vi "get_fifo.vi"(11 "FIFO":string) -> (1 "XY Graph":cluster{i32[], dbl[]}[](graph), 3 "Array":T2(array[cluster]))   [LabVIEW 2020]
panel:
  out "x/y":cdb[](array[numeric])
  out "Waveform Graph":i32[](graph)
  out "value":T1
  out "Cluster":T1
  out "rest of the binary string":string
  out "Numeric 2":u16
  in  "Numeric":u16 format="%x"
  out "Array 4":i32[](array[numeric])
  out "length 2":i32
  out "data string":string
  out "offset (0)":i32=31
  out "read buffer":string
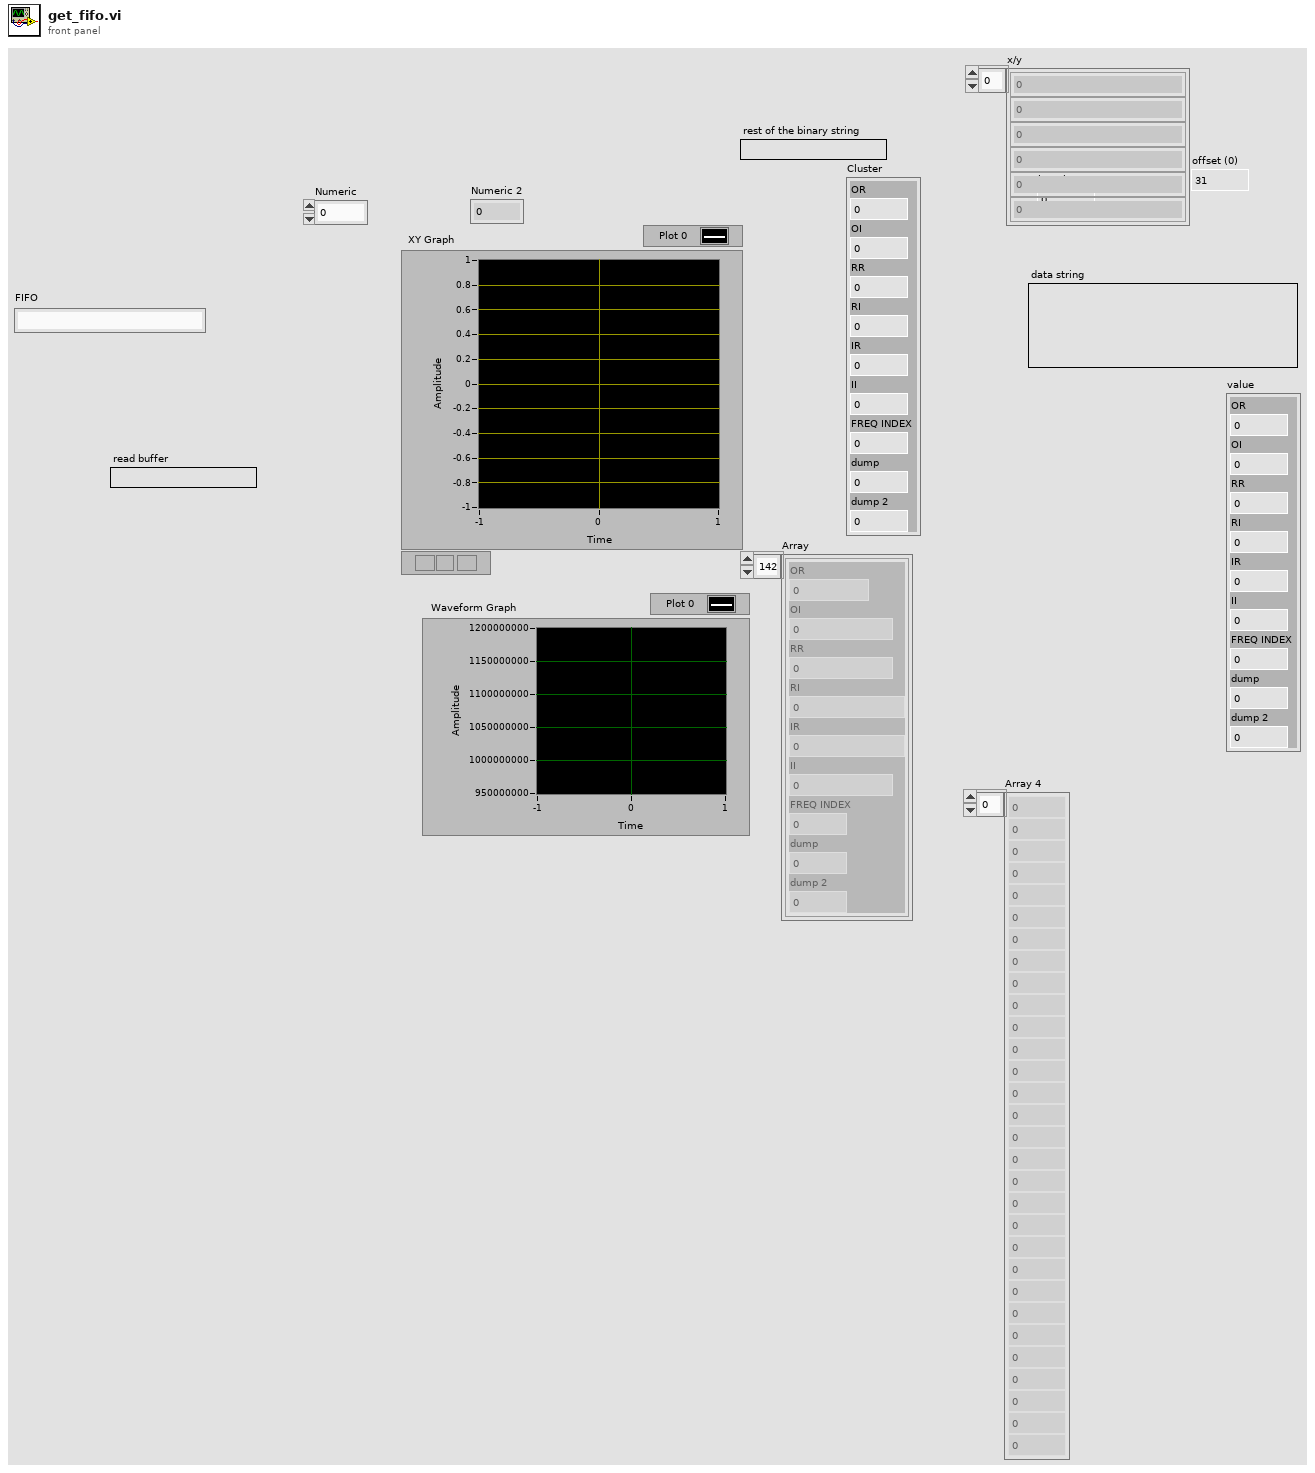
[diagram p1: front panel]
types:
  T1 = cluster{"OR":i32, "OI":i32, "RR":i32, "RI":i32, "IR":i32, "II":i32, "FREQ INDEX":u16, "dump":u16, "dump 2":u32}
  T2 = cluster{"OR":i32, "OI":i32, "RR":i32, "RI":i32, "IR":i32, "II":i32, "FREQ INDEX":u16, "dump":u16, "dump 2":u32}[]
  T3 = enum16{"big-endian, network order", "native, host order", "little-endian"}
diagram:
  w2 = 32 ("offset (0)")
  (unwired) "\u0000\u0000\u0000@\u0000\u0000\u0000\u0000l\u0002I\u0014Ü\b\u0000\u0000\u0000ÿÿÿ\u0001\u0000\u0000\u0000\u0000\u0000\u0000y\u0000\u0000\u0000@\u0000\u0000\u0000\u0000\u0006²ð/aFÿÿÿÿÿÿ\u0001\u0000\u0000\u0000\u0000\u0000\u0000Â\u0000\u0000\u0000@\u0000\u0000\u0000\u0000\u0000C!ÅP\u0000\u0000\u0000ÿÿÿ\u0001\u0000\u0000\u0000\u0000\u0000\u0000E\u0000\u0000\u0000@\u0000\u0000\u0000\u0000àb%\u001f¸£ùÿÿÿ\u0000\u0000\u0000\u0001\u0000\u0000\u0000\u0000\u0000\u0000\u0000\u0000\u0000@\u0000\u0000\u0000\u0000 y[ò@¹\u0007>\u0000\u0000\u0000\u0000\u0000\u0000\u0001\u0000\u0000\u0000\u0000\u0000\u0000p\u0000\u0000\u0000@\u0000\u0000\u0000\u0000\u0000 ÆD\u0000Üe\u0000\u0000\u0000\u0000\u0000\u0000\u0001\u0000\u0000\u0000\u0000\u0000\u0000k\u0000\u0000\u0000@\u0000\u0000\u0000\u0000 \\\u0010ðGÍ\u0001\u0000\u0000\u0000ÿÿÿ\u0001\u0000\u0000\u0000\u0000\u0000\u0000>\u0000\u0000\u0000@\u0000\u0000\u0000\u0000Ð\u0003¬\u0007ÿÿÿ\u0000\u0000\u0000\u0000\u0000\u0000\u0001\u0000\u0000\u0000\u0000\u0000\u0000\u0004\u0000\u0000\u0000@\u0000\u0000\u0000\u0000@µÝæÀ°\u001f(\u0000\u0000\u0000\u0000\u0000\u0000\u0001\u0000\u0000\u0000\u0000\u0000\u0000_\u0000\u0000\u0000@\u0000\u0000\u0000\u0000ÀO. Iï\u001f\u0000\u0000\u0000ÿÿÿ\u0001\u0000\u0000\u0000\u0000\u0000\u0000\u0000\u0000\u0000@\u0000\u0000\u0000\u0000kE \u0000±ÝB\u0000\u0000\u0000ÿÿÿ\u0001\u0000\u0000\u0000\u0000\u0000\u0000¨\u0000\u0000\u0000@\u0000\u0000\u0000\u0000À¥ã\u0000ÊÝG\u0000\u0000\u0000\u0000\u0000\u0000\u0001\u0000\u0000\u0000\u0000\u0000\u0000w\u0000\u0000\u0000@\u0000\u0000\u0000\u0000ÿÿÿÀûï\u001fÿÿÿÿÿÿ\u0001\u0000\u0000\u0000\u0000\u0000\u0000W\u0000\u0000\u0000@\u0000\u0000\u0000\u0000P«'÷äi$\u0001ÿÿÿ\u0000\u0000\u0000\u0001\u0000\u0000\u0000\u0000\u0000\u0000\u0000\u0000\u0000@\u0000\u0000\u0000\u0000 ê=(ÿÿÿÿÿÿ\u0001\u0000\u0000\u0000\u0000\u0000\u0000ì\u0000\u0000\u0000@\u0000\u0000\u0000\u0000ØøN\u0007\u0000\u001dæÒÿÿÿÿÿÿ\u0001\u0000\u0000\u0000\u0000\u0000\u0000\u0000\u0000\u0000@\u0000\u0000\u0000\u0000\u0000\u0000\u0000@/ÝÖ\u0000\u0000\u0000\u0000\u0000\u0000\u0001\u0000\u0000\u0000\u0000\u0000\u0000v\u0000\u0000\u0000@\u0000\u0000\u0000\u0000\u001aÌÂÀ7©$ÿÿÿÿÿÿ\u0001\u0000\u0000\u0000\u0000\u0000\u0000\u0018\u0000\u0000\u0000@\u0000\u0000\u0000\u0000\u0000gÊ\u0011Àm=ÿÿÿ\u0000\u0000\u0000..." ("read buffer")
  n1 = String Length(string="FIFO") -> (length=w3:i32)
  n2 = Less?(x=w3, y=w2) -> (x < y?=w1:bool)
  n3 = case shown="False" w1 {
    tunnel: "FIFO" -> [w49 _]
    tunnel: w2 -> [w48 _]
    frame False {
      w30 = 201
      w54 = T1 {"OR"=2147483647, "OI"=2147483647, "RR"=2147483647, "RI"=2147483647, "IR"=2147483647, "II"=2147483647, "FREQ INDEX"=65535, "dump"=65535, "dump 2"=2147483647}
      n4 = while {
        tunnel: w48 -> [w67]
        shift-right: [w62] -> _
        shift-left: w49 -> [w68]
        tunnel: [w64] -> w34 mode=indexing
        tunnel: [w63] -> w58 mode=indexing
        stop <- w65 stop-if-true
        n5 = Search/Split String(string=w68, offset (0)=w67) -> (substring before match=w64:string, match + rest of string=w62:string)  [unwired: 1 in, 1 out]
        n6 = String Length(string=w62) -> (length=w66:i32)
        n7 = Less?(x=w66, y=w67) -> (x < y?=w65:bool)
        n8 = String Length(string=w64) -> (length=w63:i32)
      }
      "Array 4" <- w58
      n9 = Array Size(array=w34) -> ()  [unwired: 1 out]
      n10 = Initialize Array(0 ("OR"), w30) -> (w33:i32[])
      n11 = for {
        N: w30 -> [_]
        tunnel: w34 -> [w91] mode=indexing
        tunnel: w54 -> [w94]
        tunnel: [w93] -> w52
        tunnel: [w93] -> w51 mode=indexing
        tunnel: [w89] -> w31 mode=indexing
        tunnel: [w88] -> w46 mode=indexing
        tunnel: [w85] -> w45 mode=indexing
        tunnel: [w84] -> w44 mode=indexing
        tunnel: [w83] -> w43 mode=indexing
        tunnel: [w82] -> w42 mode=indexing
        tunnel: [w86] -> w47 mode=indexing
        shift-right: [w81] -> w29
        shift-left: w33 -> [w70]
        shift-right: [w80] -> w28
        shift-left: w33 -> [w71]
        shift-right: [w79] -> w27
        shift-left: w33 -> [w72]
        shift-right: [w78] -> w26
        shift-left: w33 -> [w73]
        shift-right: [w77] -> w19
        shift-left: w33 -> [w74]
        shift-right: [w76] -> w18
        shift-left: w33 -> [w75]
        tunnel: [w69] -> w10 mode=indexing
        i -> [w69]
        n12 = Unflatten From String(type=w94, binary string=w91, data includes array or string size? (T)=FALSE, byte order (0:big-endian, network order)=T3."little-endian") -> (value=w93:T1)  [unwired: 1 in, 2 out]
        n13 = Unbundle By Name(w93) -> ("OR"=w89:i32, "OI"=w88:i32, "RR"=w85:i32, "RI"=w84:i32, "IR"=w83:i32, "II"=w82:i32, "FREQ INDEX"=w87:u16)
        n14 = To Long Integer(number=w87) -> (32bit integer=w86:i32)
        n15 = Replace Array Subset(array=w75, new element=w82, index=w86) -> (w76:i32[])
        n16 = Replace Array Subset(array=w72, new element=w85, index=w86) -> (w79:i32[])
        n17 = Replace Array Subset(array=w73, new element=w84, index=w86) -> (w78:i32[])
        n18 = Replace Array Subset(array=w74, new element=w83, index=w86) -> (w77:i32[])
        n19 = Replace Array Subset(array=w70, new element=w89, index=w86) -> (w81:i32[])
        n20 = Replace Array Subset(array=w71, new element=w88, index=w86) -> (w80:i32[])
      }
      "Cluster" <- w52
      "Array" <- w51
      "Waveform Graph" <- w31
      n21 = Flatten To String(anything=w54, prepend array or string size? (T)=FALSE, byte order (0:big-endian, network order)=T3."little-endian") -> (data string=w55:string)  [unwired: 1 in, 2 out]
      "data string" <- w55
      n22 = String Length(string=w55) -> (length=→"length 2":i32)
      n23 = Re/Im To Complex(1:w28, 2:w29) -> (0:w16:cdb[])
      n24 = Re/Im To Complex(1:w26, 2:w27) -> (0:w25:cdb[])
      n25 = Re/Im To Complex(1:w18, 2:w19) -> (0:w17:cdb[])
      n26 = Unflatten From String(type=w54, binary string=w55, data includes array or string size? (T)=FALSE, byte order (0:big-endian, network order)=T3."little-endian") -> (rest of the binary string=→"rest of the binary string":string, value=→"value":T1)  [unwired: 1 in, 1 out]
      n27 = Divide(x=w25, y=w16) -> (x/y=w24:cdb[])
      n28 = Divide(x=w17, y=w16) -> (x/y=w13:cdb[])
      "x/y" <- w13
      n29 = Bundle(w47, w45) -> (w39:cluster{i32[], i32[]})  [unwired: 1 in]
      n30 = Bundle(w47, w44) -> (w38:cluster{i32[], i32[]})  [unwired: 1 in]
      n31 = Bundle(w47, w43) -> (w37:cluster{i32[], i32[]})  [unwired: 1 in]
      n32 = Bundle(w47, w31) -> (w41:cluster{i32[], i32[]})  [unwired: 1 in]
      n33 = Bundle(w47, w46) -> (w40:cluster{i32[], i32[]})  [unwired: 1 in]
      n34 = Bundle(w47, w42) -> (w36:cluster{i32[], i32[]})  [unwired: 1 in]
      n35 = Complex To Re/Im(x + iy=w24) -> (x=w23:dbl[], y=w22:dbl[])
      n36 = Complex To Re/Im(x + iy=w13) -> (x=w12:dbl[], y=w11:dbl[])
      n37 = Complex To Re/Im(x + iy=w16) -> (x=w15:dbl[], y=w14:dbl[])
      n38 = Build Array(w41, w40, w39, w38, w37, w36) -> ()  [unwired: 1 out]
      n39 = Bundle(w10, w23) -> (w20:cluster{i32[], dbl[]})  [unwired: 1 in]
      n40 = Bundle(w10, w22) -> (w21:cluster{i32[], dbl[]})  [unwired: 1 in]
      n41 = Bundle(w10, w15) -> (w6:cluster{i32[], dbl[]})  [unwired: 1 in]
      n42 = Bundle(w10, w14) -> (w7:cluster{i32[], dbl[]})  [unwired: 1 in]
      n43 = Bundle(w10, w12) -> (w9:cluster{i32[], dbl[]})  [unwired: 1 in]
      n44 = Bundle(w10, w11) -> (w8:cluster{i32[], dbl[]})  [unwired: 1 in]
      n45 = Build Array(w6, w7, w20, w21, w9, w8) -> (→"XY Graph":cluster{i32[], dbl[]}[])
      "read buffer" <- w49
      "offset (0)" <- w48
    }
    frame True {
    }
  }
  "Numeric 2" <- "Numeric"
